vi "Kodu.vi"() -> ()   [LabVIEW 2018]
panel:
  in  "Stop":bool
  in  "length (rest) 2":i32
  in  "offset (0) 2":i32
  in  "length (rest)":i32
  in  "offset (0)":i32
  out "substring 2":string
  out "substring":string
  out "text":string
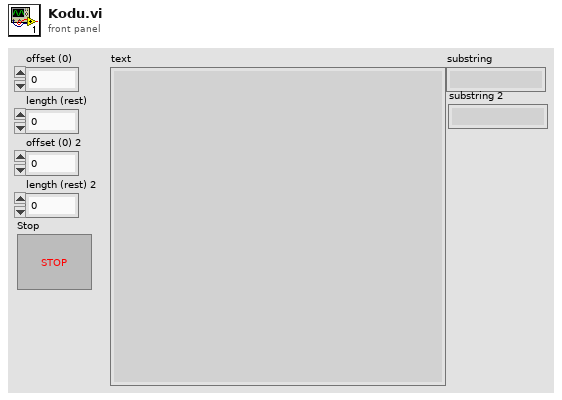
[diagram p1: front panel]
types:
  T1 = enum16{"open", "replace", "create", "open or create", "replace or create", "replace or create with confirmation"}
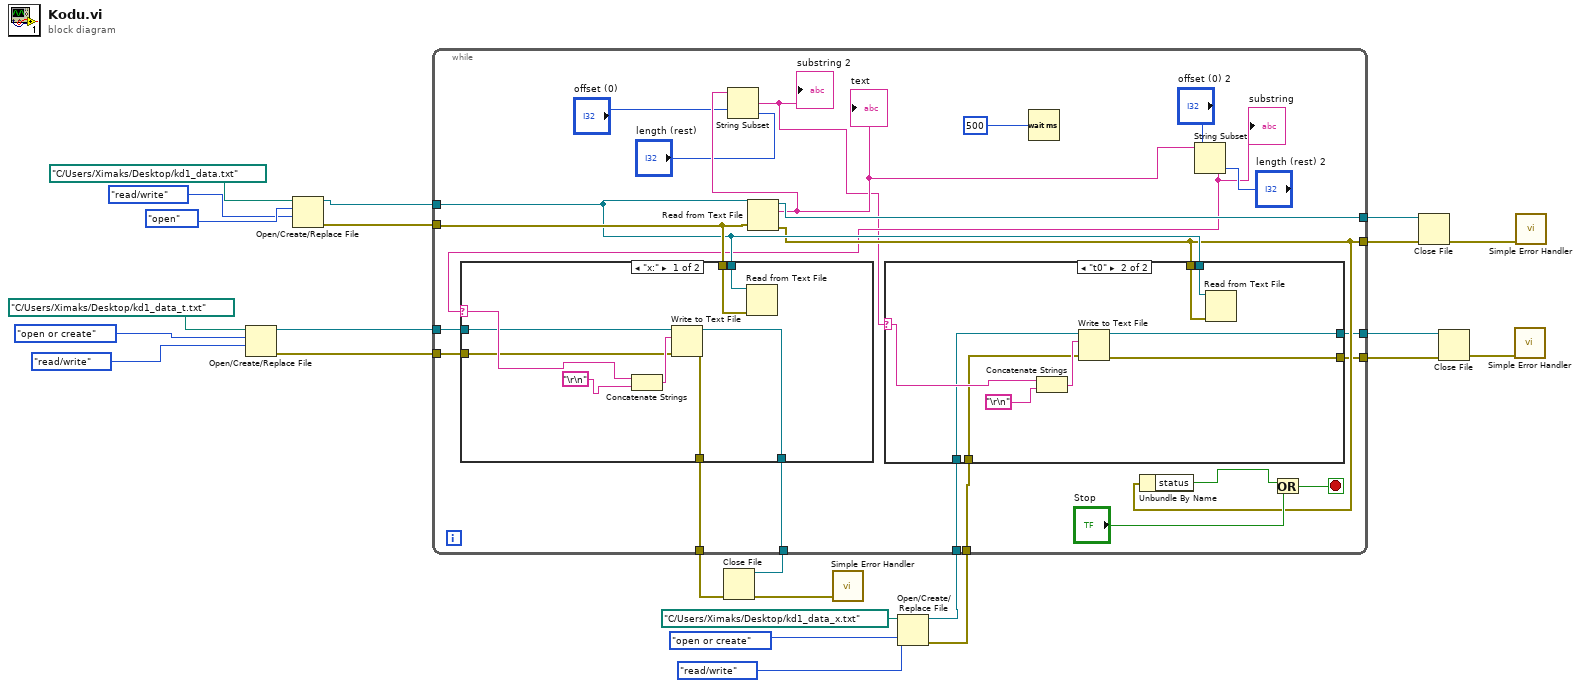
[diagram p0: block diagram]
diagram:
  n1 = Open/Create/Replace File(file path (use dialog)=path "C:/Users/Ximaks/Desktop/kd1_data_t.txt", operation (0:open)=T1."open or create", access (0:read/write)=enum16{"read/write", "read-only", "write-only"}."read/write") -> (refnum out=w10:refnum<file>, error out=w9:errorcluster)  [unwired: 3 in, 1 out]
  n2 = Open/Create/Replace File(file path (use dialog)=path "C:/Users/Ximaks/Desktop/kd1_data.txt", operation (0:open)=T1."open", access (0:read/write)=enum16{"read/write", "read-only", "write-only"}."read/write") -> (refnum out=w17:refnum<file>, error out=w18:errorcluster)  [unwired: 3 in, 1 out]
  n3 = Open/Create/Replace File(file path (use dialog)=path "C:/Users/Ximaks/Desktop/kd1_data_x.txt", operation (0:open)=T1."open or create", access (0:read/write)=enum16{"read/write", "read-only", "write-only"}."read/write") -> (refnum out=w5:refnum<file>, error out=w4:errorcluster)  [unwired: 3 in, 1 out]
  n4 = while {
    tunnel: [w47] -> w20
    tunnel: [w36] -> w19
    tunnel: w18 -> [w41]
    tunnel: w17 -> [w40]
    tunnel: [w35] -> w16
    tunnel: [w34] -> w15
    tunnel: [w33] -> w12
    tunnel: [w32] -> w11
    tunnel: w10 -> [w28]
    tunnel: w9 -> [w27]
    tunnel: w5 -> [w26]
    tunnel: w4 -> [w25]
    stop <- w39 stop-if-true
    n5 = Read from Text File(file (use dialog)=w40, error in=w41) -> (refnum out=w47:refnum<file>, text=w46:string, error out=w36:errorcluster)  [unwired: 2 in, 1 out]
    "text" <- w46
    n6 = String Subset(string=w46, offset (0)="offset (0)", length (rest)="length (rest)") -> (substring=w29:string)
    "substring 2" <- w29
    n7 = case shown="\"t0\"" w29 {
      selector: w29 -> [_ w55]
      tunnel: w40 -> [w48 w58]
      tunnel: w36 -> [w49 w57]
      tunnel: [w48 w54] -> w35
      tunnel: [w49 w53] -> w34
      tunnel: w26 -> [_ w51]
      tunnel: w25 -> [_ w50]
      frame "", Default {
      }
      frame "t0" {
        n8 = Concatenate Strings(w55, "\r\n") -> (w56:string)
        n9 = Write to Text File(file (use dialog)=w51, text=w56, error in=w50) -> (refnum out=w54:refnum<file>, error out=w53:errorcluster)  [unwired: 1 in, 1 out]
        n10 = Read from Text File(file (use dialog)=w58, error in=w57) -> ()  [unwired: 2 in, 4 out]
      }
    }
    n11 = Wait (ms)(milliseconds to wait=500) -> ()  [unwired: 1 out]
    n12 = Unbundle By Name(w36) -> ("status"=w38:bool)
    n13 = String Subset(string=w46, offset (0)="offset (0) 2", length (rest)="length (rest) 2") -> (substring=w30:string)
    "substring" <- w30
    n14 = case shown="\"x:\"" w30 {
      selector: w30 -> [w64 _]
      tunnel: w40 -> [w67 w68]
      tunnel: w41 -> [w66 w69]
      tunnel: [w63 w68] -> w33
      tunnel: [w62 w69] -> w32
      tunnel: w28 -> [w60 _]
      tunnel: w27 -> [w59 _]
      frame "x:" {
        n15 = Concatenate Strings(w64, "\r\n") -> (w65:string)
        n16 = Write to Text File(file (use dialog)=w60, text=w65, error in=w59) -> (refnum out=w63:refnum<file>, error out=w62:errorcluster)  [unwired: 1 in, 1 out]
        n17 = Read from Text File(file (use dialog)=w67, error in=w66) -> ()  [unwired: 2 in, 4 out]
      }
      frame "", Default {
      }
    }
    n18 = Or(x=w38, y="Stop") -> (x .or. y?=w39:bool)
  }
  n19 = Close File(refnum=w12, error in=w11) -> (error out=w13:errorcluster)  [unwired: 1 out]
  n20 = call <vilib>:"Simple Error Handler.vi"("error in (no error)"=w13) -> ()  [unwired: 4 in, 5 out]
  n21 = Close File(refnum=w20, error in=w19) -> (error out=w21:errorcluster)  [unwired: 1 out]
  n22 = Close File(refnum=w16, error in=w15) -> (error out=w14:errorcluster)  [unwired: 1 out]
  n23 = call <vilib>:"Simple Error Handler.vi"("error in (no error)"=w14) -> ()  [unwired: 4 in, 5 out]
  n24 = call <vilib>:"Simple Error Handler.vi"("error in (no error)"=w21) -> ()  [unwired: 4 in, 5 out]
